vi "Subscriber-2.vi"() -> ()   [LabVIEW 2015]
uses:
  <vilib>/Distrio/LabbitMQ/Channel/exchange_type_enum.ctl
  <vilib>/Distrio/LabbitMQ/Connection/Connection.lvclass
  <vilib>/Distrio/LabbitMQ/Connection/connection_parameters_cluster.ctl
  <vilib>/Platform/TimedLoop/XDataNode/timing_clust.ctl
  <vilib>/Platform/TimedLoop/XDataNode/nitl_modes.ctl
  <vilib>/Platform/TimedLoop/XDataNode/wakeup.ctl
  <vilib>/platform/TimedLoop/XDataNode/XDataNode.xnode
  <vilib>/Distrio/LabbitMQ/Queue/Queue.lvclass
  <vilib>/Distrio/LabbitMQ/Channel/Channel.lvclass
  <vilib>/Platform/TimedLoop/XDataNode/XDNodeRunTimeDep.lvlib
panel:
  in  "buttonStop":bool
  out "Received Message":string
  in  "Subscribe":bool
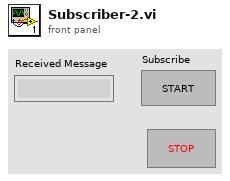
[diagram p1: front panel]
types:
  T1 = typedef "Connection.lvclass/connection_parameters_cluster.ctl" = cluster{"host name":string, "port":i32, "user name":string, "password":string, "virtual host":string}
  T2 = typedef "Channel.lvclass/exchange_type_enum.ctl" = enum16{"direct", "topic", "fanout", "headers"}
  T3 = typedef "XDNodeRunTimeDep.lvlib/timing_clust.ctl" = cluster{"Expected End [f-1]":u64, "Actual End [f-1]":u64, "Finished Late? [f-1]":bool, "Expected End [i-1]":u64, "Actual End [i-1]":u64, "Finished Late? [i-1]":bool, "Expected Start [i]":u64, "Actual Start [i]":u64, "Expected Start [f]":u64, "Actual Start [f]":u64, "Source Name":string, "Structure Name":string, "Period":i64, "Deadline":i64, "Offset":i64, "Start":i64, "Priority":i32, "Timeout":i32, "Mode":T4, "Wakeup Reason":T5, "Error":errorcluster, "Source Type":string, "Secondary Source Type":string, "Global End Time":u64, "Global Start Time":u64, "Frame Duration":u64, "Iteration Duration":u64, "Assigned CPU":i32, "I/O Scan Engine Mode":u32}
  T4 = typedef "XDNodeRunTimeDep.lvlib/nitl_modes.ctl" = enum32{"No Change", "Process missed periods, maintain original phase", "Discard missed periods, maintain original phase", "Process missed periods, ignore original phase", "Discard missed periods, ignore original phase"}
  T5 = typedef "XDNodeRunTimeDep.lvlib/wakeup.ctl" = enum32{"Normal", "Aborted", "Asynchronous wakeup", "Timing source error", "Timed loop error", "Timeout"}
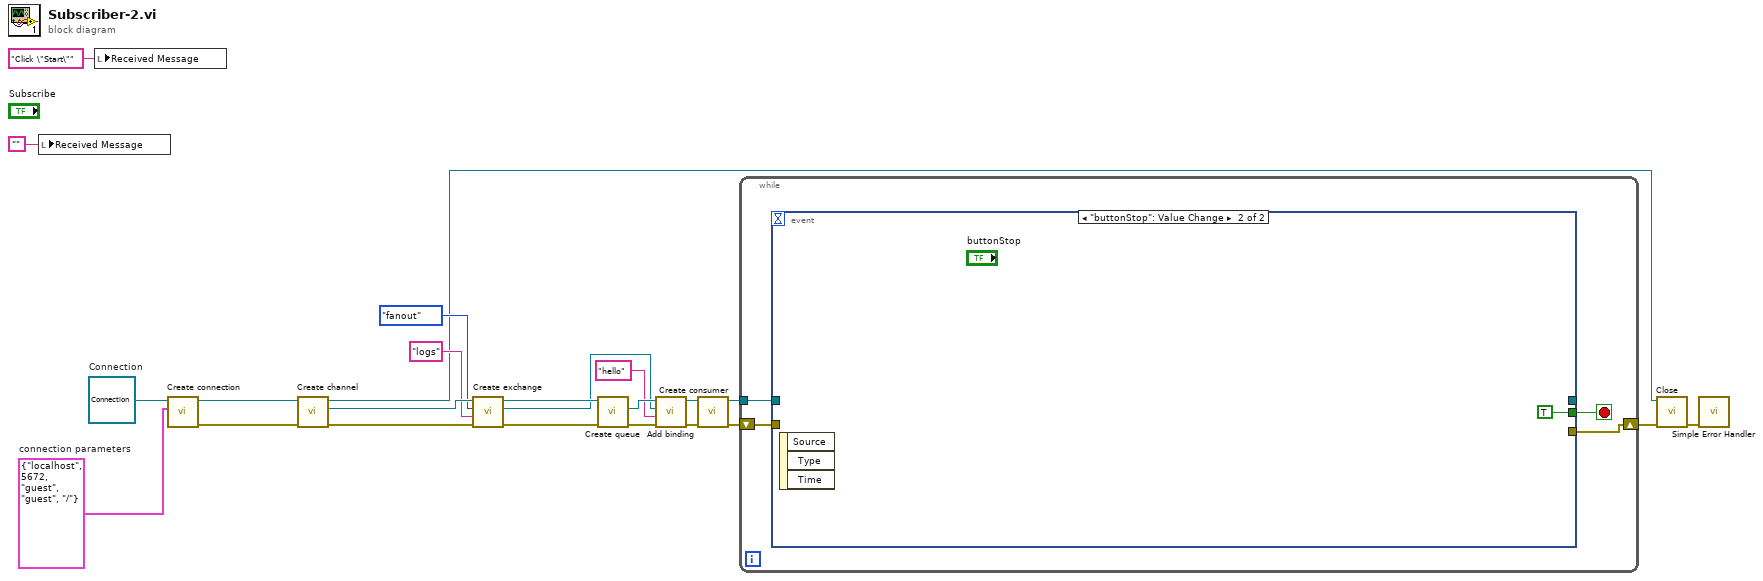
[diagram p0: block diagram]
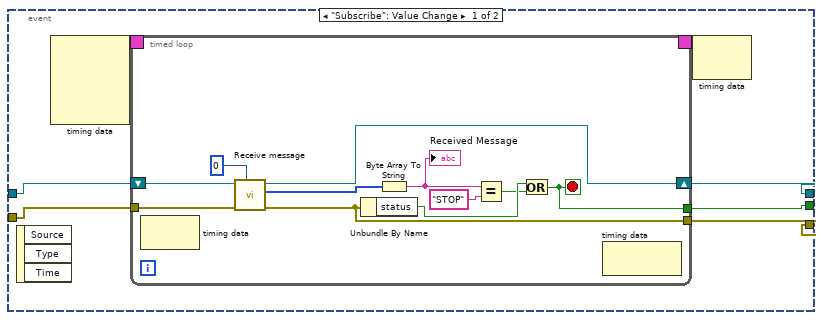
[diagram p2: hidden frame]
diagram:
  w8 = T1 {"host name"="localhost", "port"=5672, "user name"="guest", "password"="guest", "virtual host"="/"}  # connection parameters
  w9 = refnum<class "Connection.lvclass"> refnum  # Connection
  n1 = local write "Received Message"("") -> ()
  n2 = local write "Received Message"("Click \"Start\"") -> ()
  n3 = call <vilib>:"Create connection.vi"("connection parameters"=w8, "Connection in"=w9) -> ("error out"=w22:errorcluster, "Connection out"=w23:refnum<class "Connection.lvclass">)  [unwired: 8 in]
  n4 = call <vilib>:"Create channel.vi"("error in (no error)"=w22, "Connection in"=w23) -> ("error out"=w21:errorcluster, "channel"=w20:refnum<class "Channel.lvclass">, "Connection out"=w7:refnum<class "Connection.lvclass">)  [unwired: 7 in]
  n5 = call <vilib>:"Create exchange.vi"("error in (no error)"=w21, "exchange name"="logs", "exchange type"=exchange_type_enum."fanout" ("binding"), "Channel in"=w20) -> ("error out"=w19:errorcluster, "Exchange.lvclass"=w15:refnum<class "Exchange.lvclass">, "Channel out"=w18:refnum<class "Channel.lvclass">)  [unwired: 5 in]
  n6 = call <vilib>:"Create queue.vi"("error in (no error)"=w19, "Channel in"=w18) -> ("error out"=w17:errorcluster, "Queue.lvclass"=w16:refnum<class "Queue.lvclass">)  [unwired: 7 in, 1 out]
  n7 = call <vilib>:"Add binding.vi"("error in (no error)"=w17, "binding key"="hello" ("routing key"), "Exchange.lvclass"=w15, "Consumer in"=w16) -> ("error out"=w13:errorcluster, "Consumer out"=w12:refnum<class "Queue.lvclass">)  [unwired: 6 in]
  n8 = call <vilib>:"Create consumer.vi"("error in (no error)"=w13, "Queue in"=w12) -> ("error out"=w4:errorcluster, "Queue out"=w5:refnum<class "Queue.lvclass">)  [unwired: 8 in]
  n9 = while {
    tunnel: w5 -> [w27]
    shift-right: [w25] -> w1
    shift-left: w4 -> [w26]
    stop <- w24 stop-if-true
    n10 = event shown="[1] \"buttonStop\": Value Change" {
      selector: _ -> [_ _]
      dyn-events: _ -> [_ _]
      timeout: _ -> [_ _]
      tunnel: w27 -> [w34 _]
      tunnel: w26 -> [w33 _]
      tunnel: [w32 _] -> _
      tunnel: [w30 TRUE] -> w24
      tunnel: [w31 _] -> w25
      event "Subscribe": Value Change {
        n11 = event-data() -> ()  [unwired: 1 in, 3 out]
        n12 = node-c288() -> (w29:T3)  [unwired: 4 in]
        n13 = timed-loop {
          tunnel: w33 -> [w43]
          shift-right: [w42] -> w32
          shift-left: w34 -> [w44]
          tunnel: [w37] -> w31
          tunnel: [w36] -> w30
          timing: w29 -> [_]
          timing-out: [_] -> w28
          stop <- w36 stop-if-true
          n14 = node-c288() -> ()  [unwired: 1 in, 1 out]
          n15 = call <vilib>:"Receive message.vi"("millisecondsTimeout"=0, "error in (no error)"=w43, "Consumer in"=w44) -> ("error out"=w37:errorcluster, "message body"=w45:u8[], "Consumer out"=w42:refnum<class "Queue.lvclass">)  [unwired: 3 in, 3 out]
          n16 = Unbundle By Name(w37) -> ("status"=w39:bool)
          n17 = Byte Array To String(unsigned byte array=w45) -> (string=w40:string)
          "Received Message" <- w40
          n18 = Equal?(x=w40, y="STOP") -> (x = y?=w38:bool)
          n19 = Or(x=w39, y=w38) -> (x .or. y?=w36:bool)
          n20 = node-c288() -> ()  [unwired: 1 in, 1 out]
        }
        n21 = node-c288(w28) -> ()  [unwired: 1 out]
      }
      event "buttonStop": Value Change {
        n22 = event-data() -> ()  [unwired: 1 in, 3 out]
      }
    }
  }
  n23 = call <vilib>:"Close.vi"("error in (no error)"=w1, "Connection in"=w7) -> ("error out"=w6:errorcluster)  [unwired: 8 in, 1 out]
  n24 = call <vilib>:"Simple Error Handler.vi"("error in (no error)"=w6) -> ()  [unwired: 4 in, 5 out]
